vi "ActuationTest.vi"(8 "TNom":i32=-130, 9 "Cycle":i32=5, 11 "Output base directory":path=path "E:/LTM Tests") -> ()   [LabVIEW 2024]
uses:
  <userlib>/_OpenG.lib/file/file.llb/openg_file.lvlib
panel:
  in  "Path to Actuation Script":path=path "C:/Users/dpl/OneDrive - Aberystwyth University/Documents/GitHub/Enfys-OBEGSE/ob_egse/egse.py"
  in  "Path to Python EXE":path=path "C:/ProgramData/anaconda3/python.exe"
  in  "Video Duration (min)":dbl=2.5 format="%#_13g"
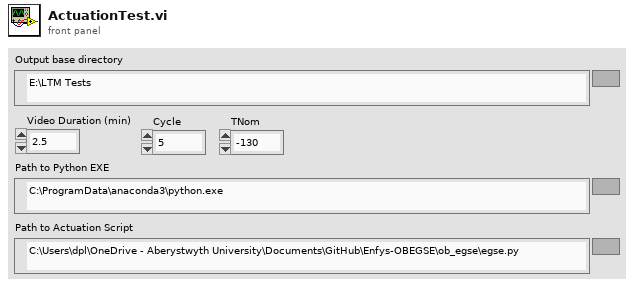
[diagram p1: front panel]
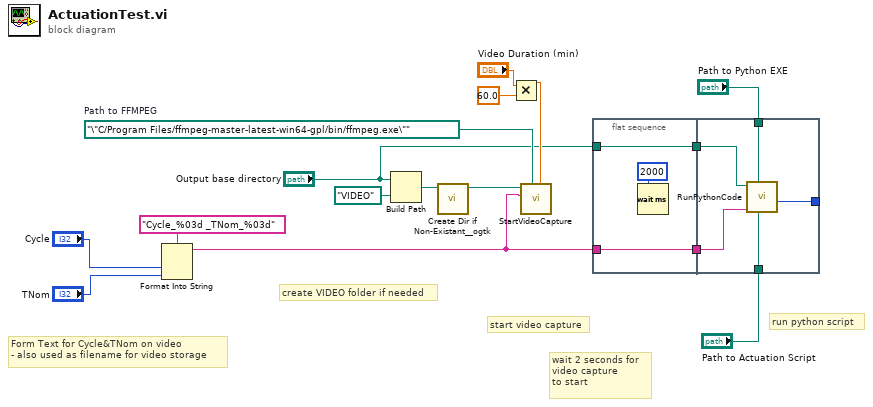
[diagram p0: block diagram]
diagram:
  w12 = path "/\"C/Program Files/ffmpeg-master-latest-win64-gpl/bin/ffmpeg.exe\""  # Path to FFMPEG
  # "create VIDEO folder if needed"
  # "run python script"
  # "wait 2 seconds for \nvideo capture \nto start"
  # "start video capture"
  # "Form Text for Cycle&TNom on video\n- also used as filename for video storage"
  n1 = Format Into String(format string="Cycle_%03d _TNom_%03d", "Cycle", "TNom") -> (resulting string=w7:string)  [unwired: 2 in, 1 out]
  n2 = Build Path(base path="Output base directory", name or relative path=path "VIDEO") -> (appended path=w2:path)
  n3 = call <userlib>:"Create Dir if Non-Existant__ogtk.vi"("Directory Path"=w2) -> ("dup Directory Path"=w1:path)  [unwired: 8 in, 2 out]
  n4 = Multiply(x="Video Duration (min)", y=60.0) -> (x*y=w15:dbl)
  n5 = call "StartVideoCapture.vi"("Output Directory"=w1, "SaveFile"=w7, "Path to FFMPEG"=w12, 5:w15) -> ()  [unwired: 5 in, 2 out]
  n6 = flat-sequence {
    tunnel: w7 -> [w18]
    tunnel: "Output base directory" -> [w19]
    tunnel: [w19] -> w4
    tunnel: [w18] -> w3
    tunnel: "Path to Python EXE" -> [w22]
    tunnel: "Path to Actuation Script" -> [w21]
    tunnel: w4 -> [w24]
    tunnel: w3 -> [w23]
    tunnel: [w20] -> _
    frame #0 {
      n7 = Wait (ms)(milliseconds to wait=u32 2000) -> ()  [unwired: 1 out]
    }
    frame #1 {
      n8 = call "RunPythonCode.vi"("Path to Actuation Script"=w21, "COM Port"=w22, "error in (no error)"=w23, "Output base directory"=w24) -> ("return code"=w20:i32)  [unwired: 6 in, 1 out]
    }
  }
